vi "Count_if_Subtrack_Is_Enough_for_Cost_F()-2.vi"(3 "[IN] Minimal Subtrack Length \n(Points without problems) for\nMaking Desicion":i32, 4 "[IN] Index of Problem \nPoint Inside Track":i32, 5 "[IN] Dot Statuses in Track":i16[](array[numeric])) -> (1 "[OUT] Index of Last \nPoint in Track":i32, 2 "[OUT] It's enough to make\nconclusion using subtrack":bool)   [LabVIEW 2013]
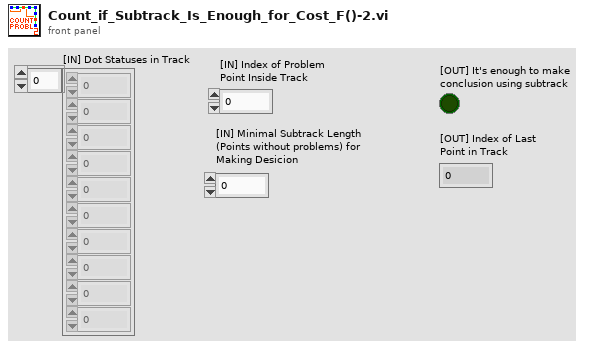
[diagram p1: front panel]
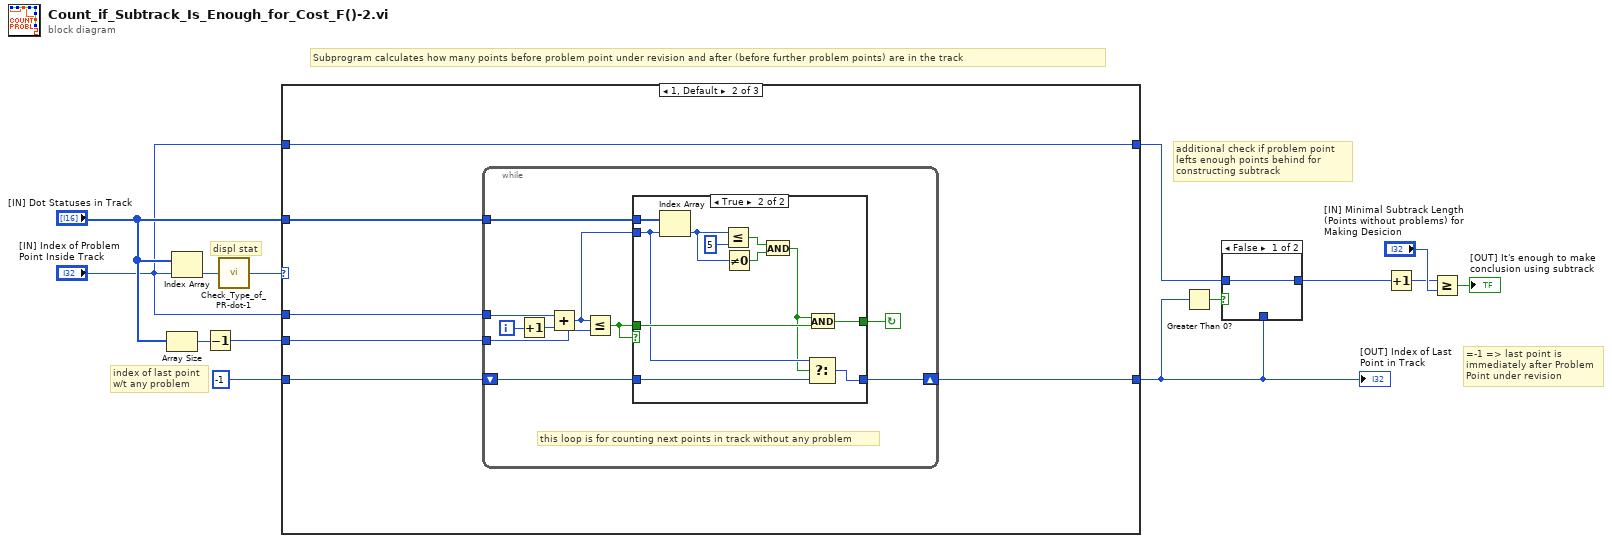
[diagram p0: block diagram]
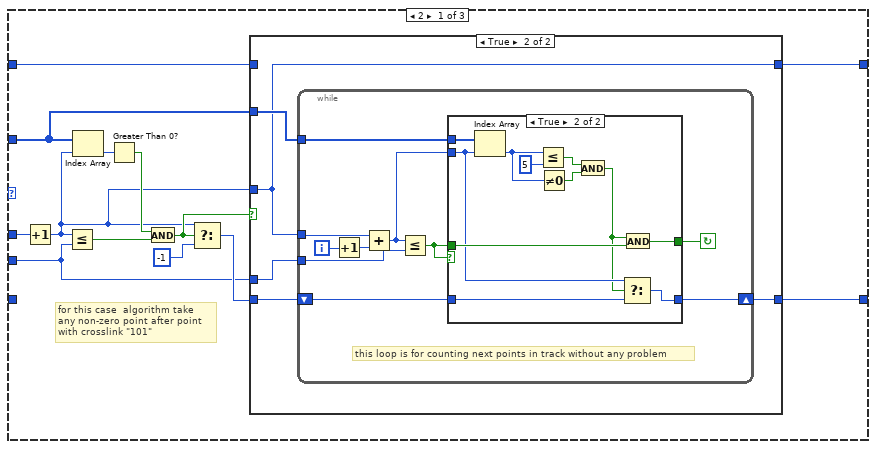
[diagram p2: hidden frame]
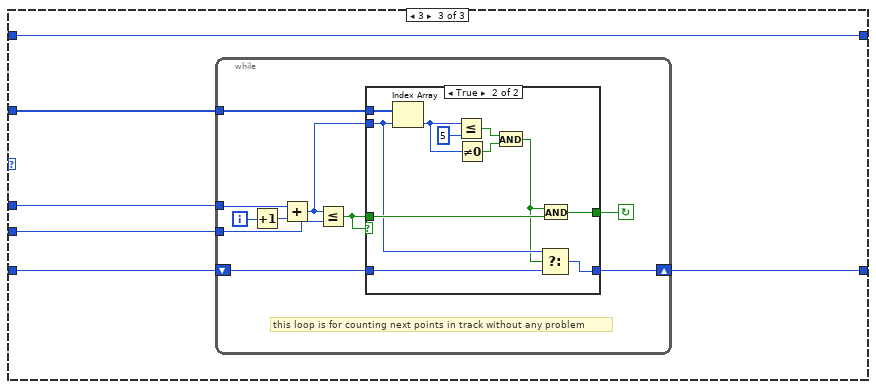
[diagram p6: hidden frame]
diagram:
  # "displ stat"
  # "additional check if problem point \nlefts enough points behind for \nconstructing subtrack"
  # "=-1 => last point is\nimmediately after Problem \nPoint under revision"
  # "Subprogram calculates how many points before problem point under revision and after (before further problem points) are in the track"
  # "index of last point\nw/t any problem"
  n1 = Array Size(array="[IN] Dot Statuses in Track") -> (size(s)=w14:i32)
  n2 = Index Array(array="[IN] Dot Statuses in Track", index="[IN] Index of Problem \nPoint Inside Track") -> (element=w4:i16)
  n3 = Decrement(x=w14) -> (x-1=w13:i32)
  n4 = call "Check_Type_of_PR-dot-1.vi"("[IN] dot status"=w4) -> ("[OUT] Type of\nproblem dot"=w3:i32)
  n5 = case shown="1, Default" w3 {
    tunnel: w13 -> [w17 w63 w90]
    tunnel: -1 -> [_ w62 w89]
    tunnel: [w18 w61 w88] -> w6
    tunnel: "[IN] Dot Statuses in Track" -> [w19 w60 w92]
    tunnel: "[IN] Index of Problem \nPoint Inside Track" -> [w27 w59 w91]
    tunnel: "[IN] Index of Problem \nPoint Inside Track" -> [w15 w58 w87]
    tunnel: [w16 w58 w87] -> w1
    frame 2 {
      # "for this case  algorithm take\nany non-zero point after point\nwith crosslink \"101\""
      n6 = Increment(x=w27) -> (x+1=w20:i32)
      n7 = Less Or Equal?(x=w20, y=w17) -> (x <= y?=w25:bool)
      n8 = Index Array(array=w19, index=w20) -> (element=w26:i16)
      n9 = Greater Than 0?(x=w26) -> (x > 0?=w24:bool)
      n10 = And(x=w24, y=w25) -> (x .and. y?=w22:bool)
      n11 = Select(t=w20, s=w22, f=-1) -> (s? t:f=w21:i32)
      n12 = case shown="True" w22 {
        tunnel: w21 -> [w29 w34]
        tunnel: w20 -> [_ w30]
        tunnel: w19 -> [_ w33]
        tunnel: [w29 w32] -> w18
        tunnel: w17 -> [_ w31]
        tunnel: [w28 w30] -> w16
        tunnel: w15 -> [w28 _]
        frame False {
        }
        frame True {
          n13 = while {
            tunnel: w31 -> [w42]
            tunnel: w30 -> [w35]
            tunnel: w33 -> [w41]
            shift-right: [w36] -> w32
            shift-left: w34 -> [w37]
            i -> [w44]
            stop <- w38 continue-if-true
            # "this loop is for counting next points in track without any problem"
            n14 = Increment(x=w44) -> (x+1=w43:i32)
            n15 = Add(x=w35, y=w43) -> (x+y=w40:i32)
            n16 = Less Or Equal?(x=w40, y=w42) -> (x <= y?=w39:bool)
            n17 = case shown="True" w39 {
              tunnel: w41 -> [_ w57]
              tunnel: w40 -> [_ w48]
              tunnel: w39 -> [w46 w51]
              tunnel: [w46 w52] -> w38
              tunnel: w37 -> [w45 w49]
              tunnel: [w45 w50] -> w36
              frame False {
                # "it's last point in subtrack"
              }
              frame True {
                n18 = Index Array(array=w57, index=w48) -> (element=w55:i16)
                n19 = Less Or Equal?(x=w55, y=i16 5) -> (x <= y?=w54:bool)
                n20 = Not Equal To 0?(x=w55) -> (x != 0?=w53:bool)
                n21 = And(x=w54, y=w53) -> (x .and. y?=w47:bool)
                n22 = Select(t=w48, s=w47, f=w49) -> (s? t:f=w50:i32)
                n23 = And(x=w47, y=w51) -> (x .and. y?=w52:bool)
              }
            }
          }
        }
      }
    }
    frame 1, Default {
      n24 = while {
        tunnel: w63 -> [w71]
        tunnel: w59 -> [w64]
        tunnel: w60 -> [w70]
        shift-right: [w65] -> w61
        shift-left: w62 -> [w66]
        i -> [w73]
        stop <- w67 continue-if-true
        # "this loop is for counting next points in track without any problem"
        n25 = Increment(x=w73) -> (x+1=w72:i32)
        n26 = Add(x=w64, y=w72) -> (x+y=w69:i32)
        n27 = Less Or Equal?(x=w69, y=w71) -> (x <= y?=w68:bool)
        n28 = case shown="True" w68 {
          tunnel: w70 -> [_ w86]
          tunnel: w69 -> [_ w77]
          tunnel: w68 -> [w75 w80]
          tunnel: [w75 w81] -> w67
          tunnel: w66 -> [w74 w78]
          tunnel: [w74 w79] -> w65
          frame False {
            # "it's last point in subtrack"
          }
          frame True {
            n29 = Index Array(array=w86, index=w77) -> (element=w84:i16)
            n30 = Less Or Equal?(x=w84, y=i16 5) -> (x <= y?=w83:bool)
            n31 = Not Equal To 0?(x=w84) -> (x != 0?=w82:bool)
            n32 = And(x=w83, y=w82) -> (x .and. y?=w76:bool)
            n33 = Select(t=w77, s=w76, f=w78) -> (s? t:f=w79:i32)
            n34 = And(x=w76, y=w80) -> (x .and. y?=w81:bool)
          }
        }
      }
    }
    frame 3 {
      n35 = while {
        tunnel: w90 -> [w100]
        tunnel: w91 -> [w93]
        tunnel: w92 -> [w99]
        shift-right: [w94] -> w88
        shift-left: w89 -> [w95]
        i -> [w102]
        stop <- w96 continue-if-true
        # "this loop is for counting next points in track without any problem"
        n36 = Increment(x=w102) -> (x+1=w101:i32)
        n37 = Add(x=w93, y=w101) -> (x+y=w98:i32)
        n38 = Less Or Equal?(x=w98, y=w100) -> (x <= y?=w97:bool)
        n39 = case shown="True" w97 {
          tunnel: w99 -> [_ w115]
          tunnel: w98 -> [_ w106]
          tunnel: w97 -> [w104 w109]
          tunnel: [w104 w110] -> w96
          tunnel: w95 -> [w103 w107]
          tunnel: [w103 w108] -> w94
          frame False {
            # "it's last point in subtrack"
          }
          frame True {
            n40 = Index Array(array=w115, index=w106) -> (element=w113:i16)
            n41 = Less Or Equal?(x=w113, y=i16 5) -> (x <= y?=w112:bool)
            n42 = Not Equal To 0?(x=w113) -> (x != 0?=w111:bool)
            n43 = And(x=w112, y=w111) -> (x .and. y?=w105:bool)
            n44 = Select(t=w106, s=w105, f=w107) -> (s? t:f=w108:i32)
            n45 = And(x=w105, y=w109) -> (x .and. y?=w110:bool)
          }
        }
      }
    }
  }
  "[OUT] Index of Last \nPoint in Track" <- w6
  n46 = Greater Than 0?(x=w6) -> (x > 0?=w8:bool)
  n47 = case shown="False" w8 {
    tunnel: w1 -> [w116 _]
    tunnel: [w116 w117] -> w7
    tunnel: w6 -> [_ w117]
    frame False {
    }
    frame True {
    }
  }
  n48 = Increment(x=w7) -> (x+1=w9:i32)
  n49 = Greater Or Equal?(x=w9, y="[IN] Minimal Subtrack Length \n(Points without problems) for\nMaking Desicion") -> (x >= y?=→"[OUT] It's enough to make\nconclusion using subtrack":bool)
